vi "ResetIOMerge.vi"   [LabVIEW 2020]
doc: "Resets the state, clears the data path, and clears any error conditions for the I/O items. This node also resets any pipeline stages and counters for the I/O item."
uses:
  <vilib>/eio/EIOGrowableMethodNode/genericMethod/EIOGrowableMethodNode.xnode
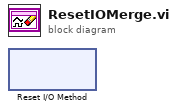
[diagram p0: block diagram]
diagram:
  n1 = xnode "Reset I/O Method"() -> ()  [unwired: 1 in, 1 out]
